vi "Async VI Control_Wait on Start Trigger.vi"(8 "error in (no error)":errorcluster, 11 "Name":string) -> (0 "error out":errorcluster, 3 "notification":bool)   [LabVIEW 2021, in "CANOpen Addon Engine.lvlib"]
uses:
  CANOpen Addon Engine.lvlib
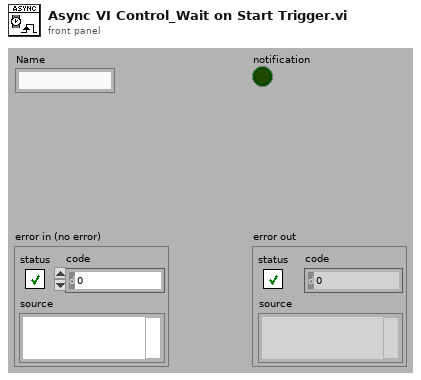
[diagram p1: front panel]
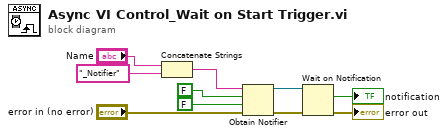
[diagram p0: block diagram]
diagram:
  n1 = Concatenate Strings("Name", "_Notifier" ("name (unnamed)")) -> (w4:string)
  n2 = Obtain Notifier(name (unnamed)=w4, notification data type=FALSE, create if not found? (T)=FALSE, error in (no error)="error in (no error)") -> (notifier out=w9:refnum<notifier>, error out=w10:errorcluster)  [unwired: 1 out]
  n3 = Wait on Notification(notifier=w9, error in (no error)=w10) -> (notification=→"notification":bool, error out=→"error out":errorcluster)  [unwired: 2 in, 2 out]
